vi "Activate DUT.vi"(8 "error in (no error)":errorcluster, 10 "DUT (\"DUT1\")":string="DUT1", 11 "VISA resource name":refnum<visa-resource-name>) -> (0 "error out":errorcluster, 3 "VISA resource name out":refnum<visa-resource-name>)   [LabVIEW 2015, in "Rohde&Schwarz CMXP Base.lvlib"]
doc: "Activates the DUT with the specified name for usage in the test environment.\n\nAttribute:\nRSCMXPBASE_ATTR_DUT_ACTIVATE\n\nRemote-control command:\nACTivate:DUT"
uses:
  <instrlib>/Rohde&Schwarz CMXP Base/Rohde&Schwarz CMXP Base.lvlib
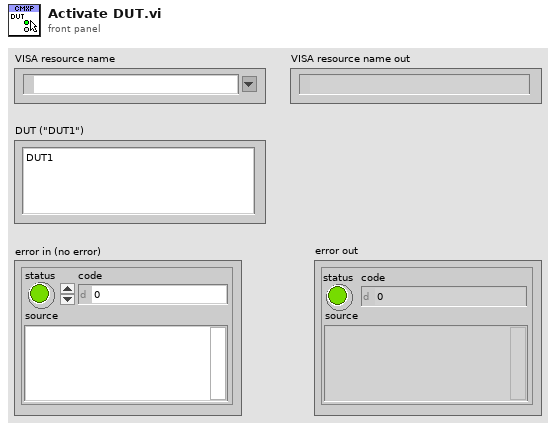
[diagram p1: front panel]
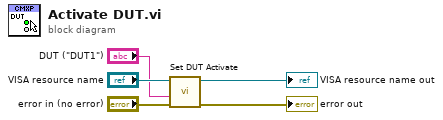
[diagram p0: block diagram]
diagram:
  n1 = call "Set DUT Activate"("error in (no error)"="error in (no error)", "DUT Activate ()"="DUT (\"DUT1\")", "instrument handle"="VISA resource name") -> ("error out"=→"error out":errorcluster, "instrument handle out"=→"VISA resource name out":refnum<visa-resource-name>)  [unwired: 7 in]
